vi "sine 3d plotter.vi"() -> ()   [LabVIEW 2020]
uses:
  <vilib>/Math Plots/3D Math Plots/3D Surface/3D Surface XCtrl/3D Surface.xctl
  <vilib>/Math Plots/3D Math Plots/3D Surface/3D Surface Datatype/Public/Plot Helper (Vector).vi
  <vilib>/Analysis/NI_AALBase.lvlib
  <vilib>/Math Plots/3D Math Plots/3D Surface/3D Surface Datatype/3D Surface Datatype.lvclass
panel:
  in  "Numeric":dbl format="%#_13g"
  out "Intensity Graph":dbl[][](graph)
  out "3D Surface":refnum<class "3D Plot Datatype.lvclass">[](xcontrol)
  out "Waveform Graph":dbl[](graph)
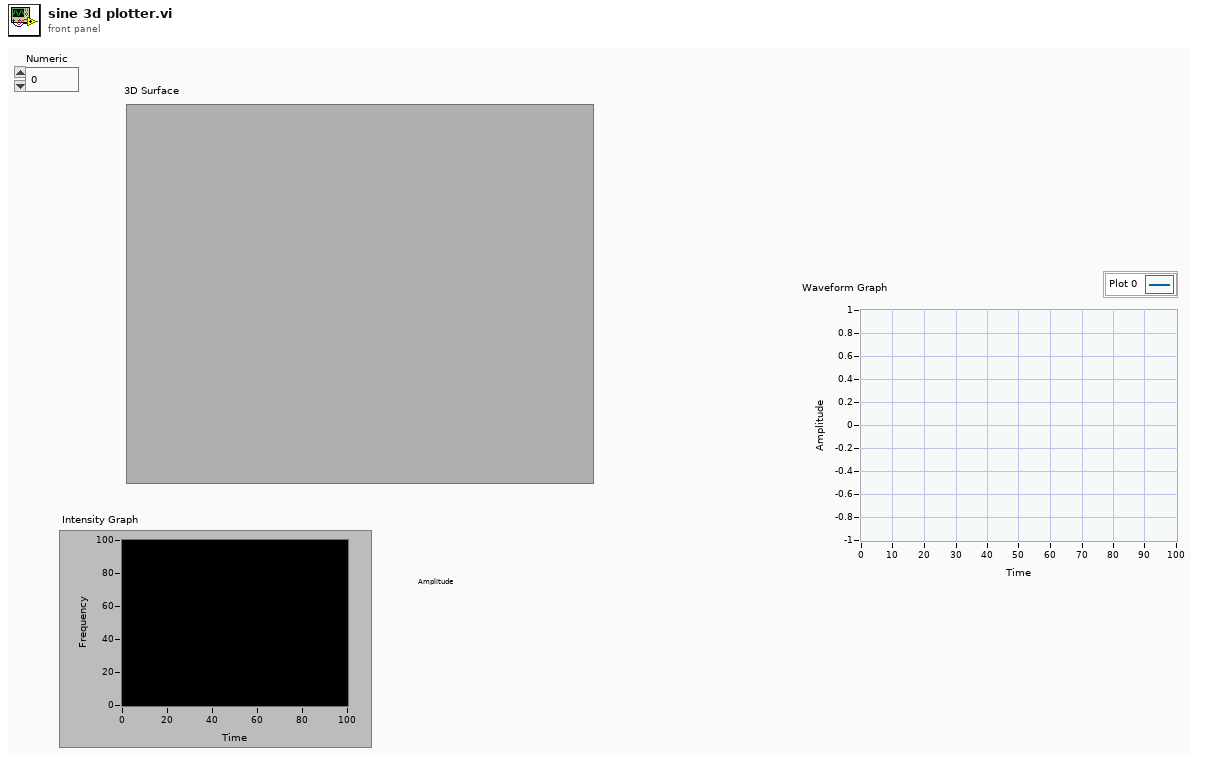
[diagram p1: front panel]
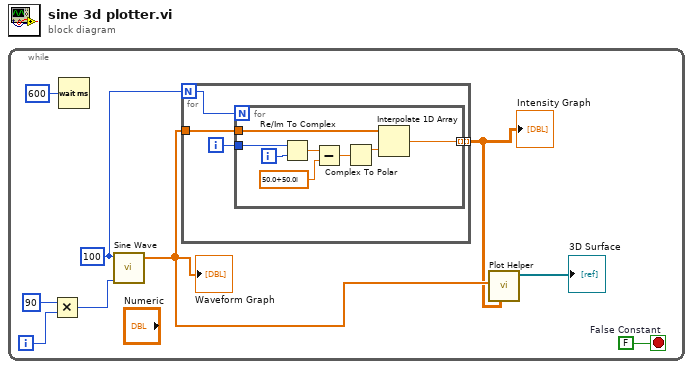
[diagram p0: block diagram]
diagram:
  n1 = while {
    i -> [w2]
    stop <- w5 stop-if-true
    w5 = FALSE  # False Constant
    w9 = 100 ("samples")
    n2 = Multiply(x=90, y=w2) -> (x*y=w8:i32)
    n3 = Wait (ms)(milliseconds to wait=u32 600) -> ()  [unwired: 1 out]
    n4 = call <vilib>:"Sine Wave.vi"("samples"=w9, "phase in"=w8) -> ("sine wave"=w3:dbl[])  [unwired: 3 in, 2 out]
    "Waveform Graph" <- w3
    n5 = for {
      N: w9 -> [w12]
      tunnel: [w11] -> w1 mode=indexing
      tunnel: w3 -> [w10]
      i -> [w13]
      n6 = for {
        N: w12 -> [_]
        tunnel: w13 -> [w20]
        tunnel: [w15] -> w11 mode=indexing
        tunnel: w10 -> [w14]
        i -> [w21]
        n7 = Re/Im To Complex(1:w21, 2:w20) -> (0:w19:cdb)
        n8 = Subtract(x=w19, y=cdb 50.0+50.0i) -> (x-y=w18:cdb)
        n9 = Complex To Polar(r * e^(i*theta)=w18) -> (r=w17:dbl)  [unwired: 1 out]
        n10 = Interpolate 1D Array(1:w17, 2:w14) -> (0:w15:dbl)
      }
    }
    "Intensity Graph" <- w1
    n11 = call-poly <vilib>:"Plot Helper.vi"("z matrix"=w1, "x vector"=w3) -> ("3D Plot lvclass Array out"=→"3D Surface":refnum<class "3D Plot Datatype.lvclass">[])  [unwired: 4 in, 5 out]
  }
